vi "Save text file.vi"(8 "error in (no error)":errorcluster, 10 "Data":dbl, 11 "TDMS in":refnum<class "TDMS.lvclass">) -> (0 "error out":errorcluster, 3 "TDMS out":refnum<class "TDMS.lvclass">)   [LabVIEW 2020, in "TDMS.lvlib" / "TDMS.lvclass"]
uses:
  TDMS.lvclass
  Text Actor/Text Actor/Text Actor.lvclass
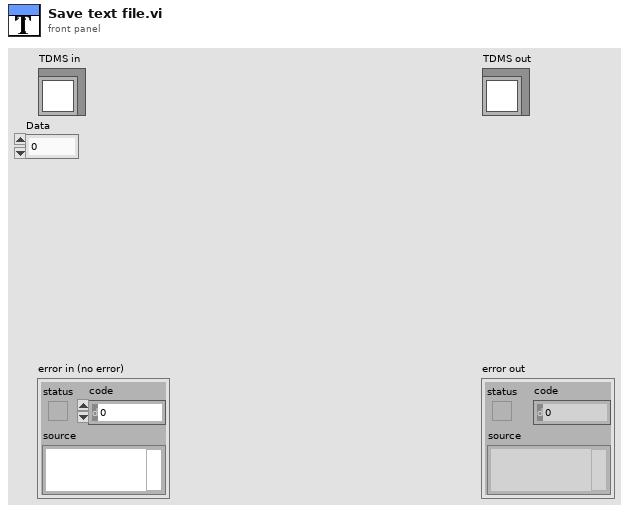
[diagram p1: front panel]
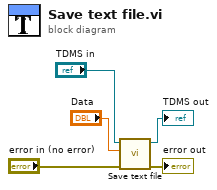
[diagram p0: block diagram]
diagram:
  n1 = call-parent "Save text file.vi"("error in (no error)"="error in (no error)", "Data"="Data", "Text Actor in"="TDMS in") -> ("error out"=→"error out":errorcluster, "Text Actor out"=→"TDMS out":refnum<class "TDMS.lvclass">)  [unwired: 7 in]
